vi "MovableControl.vi"() -> ()   [LabVIEW 2019]
uses:
  <vilib>/Utility/miscctls.llb/LVPositionTypeDef.ctl
panel:
  in  "Movable":bool
  # "我的拖拽太快不會壞掉ㄛ"
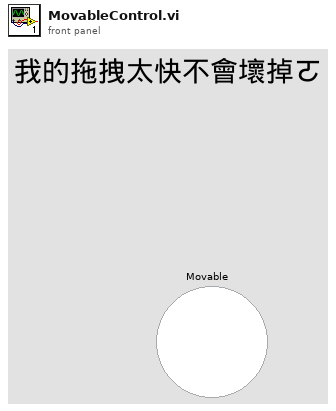
[diagram p1: front panel]
types:
  T1 = typedef "LVPositionTypeDef.ctl" = cluster{"Left":i32, "Top":i32}
  T2 = typedef "LVPoint32TypeDef.ctl" = cluster{"Horizontal":i32, "Vertical":i32}
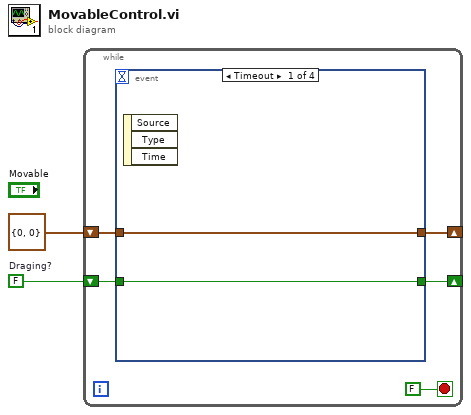
[diagram p0: block diagram]
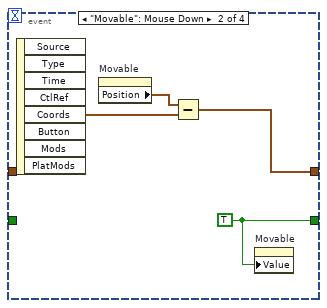
[diagram p2: hidden frame]
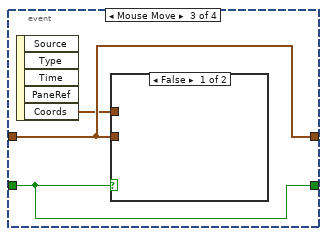
[diagram p3: hidden frame]
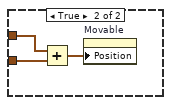
[diagram p4: hidden frame]
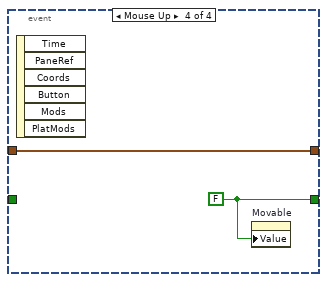
[diagram p5: hidden frame]
diagram:
  w2 = FALSE  # Draging?
  n1 = while {
    shift-right: [w6] -> _
    shift-left: w2 -> [w7]
    shift-right: [w4] -> _
    shift-left: T1 {"Left"=0, "Top"=0} ("Position") -> [w3]
    stop <- FALSE stop-if-true
    n2 = event shown="[0] Timeout" {
      selector: _ -> [_ _ _ _]
      dyn-events: _ -> [_ _ _ _]
      timeout: _ -> [_ _ _ _]
      tunnel: w7 -> [w9 _ w15 _]
      tunnel: [w9 w13 w15 w21] -> w6
      tunnel: [w8 w10 w16 w20] -> w4
      tunnel: w3 -> [w8 _ w16 w20]
      event Timeout {
        n3 = event-data() -> ()  [unwired: 1 in, 3 out]
      }
      event "Movable": Mouse Down {
        w13 = TRUE ("Draging?")
        n4 = event-data() -> ("Coords"=w11:T2)  [unwired: 1 in, 7 out]
        n5 = property on="Movable" class="Bool (strict)"() -> ("Position"=w12:T1)  [unwired: 2 in, 2 out]
        n6 = Subtract(x=w12, y=w11) -> (x-y=w10:T1)
        n7 = property on="Movable" class="Bool (strict)"("Value"=w13) -> ()  [unwired: 2 in, 2 out]
      }
      event Mouse Move {
        n8 = event-data() -> ("Coords"=w14:T2)  [unwired: 1 in, 4 out]
        n9 = case shown="False" w15 {
          tunnel: w16 -> [_ w18]
          tunnel: w14 -> [_ w19]
          frame False {
          }
          frame True {
            n10 = Add(x=w19, y=w18) -> (x+y=w17:T2)
            n11 = property on="Movable" class="Bool (strict)"("Position"=w17) -> ()  [unwired: 2 in, 2 out]
          }
        }
      }
      event Mouse Up {
        w21 = FALSE ("Draging?")
        n12 = event-data() -> ()  [unwired: 1 in, 6 out]
        n13 = property on="Movable" class="Bool (strict)"("Value"=w21) -> ()  [unwired: 2 in, 2 out]
      }
    }
  }
